vi "PDF Welding.vi"(0 "configuration file path":path caption="配置文件的路径", 1 "PDF Welding msic inf":T1) -> ()   [LabVIEW 2018]
uses:
  Ctl.xio/PDF Welding msic ctl.ctl
  SubVIS.xio/DataSocket/DataSocket_Tags.ctl
  Ctl.xio/part type.ctl
  SubVIS.xio/Creat Write List VI's/DefCtrl/Station.ctl
  SubVIS.xio/DataSocket/Write PLC Vars/Write Bool Var in.vi
  <vilib>/Utility/file.llb/Read From Spreadsheet File (string).vi
  SubVIS.xio/DataSocket/Write PLC Vars/Write String Var in.vi
  SubVIS.xio/DataSocket/Read PLC Vars/Read Bool Var.vi
  SubVIS.xio/DataSocket/Read PLC Vars/Read U32 Var.vi
  SubVIS.xio/DataSocket/Write PLC Vars/Write Dbl Var in.vi
  SubVIS.xio/Hopper car inf/Curing inf.vi
panel:
  in  "SQL information":string
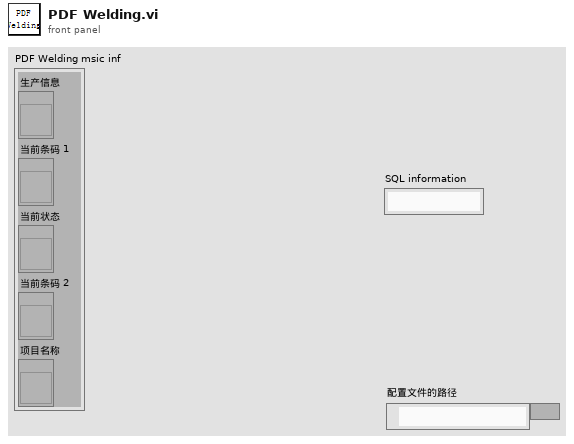
[diagram p1: front panel]
types:
  T1 = cluster{"生产信息":refnum<vi>, "当前条码 1":refnum<vi>, "当前状态":refnum<vi>, "当前条码 2":refnum<vi>, "项目名称":refnum<vi>}
  T2 = typedef "Station.ctl" = enum16{"粗切工位", "热处理工位", "精切工位", "PDF焊接工位", "打凹点预载力工位", "收卷工位", "EOL工位"}
  T3 = typedef "PDF Welding msic ctl.ctl" = cluster{"configuration file path":path, "DsOut":T4[], "Hopper car information":cluster{"Hopper car code":string, "Hopper car No":string, "plate No":string}, "pallet.produced number":i32, "SQL information":string, "Serial number":i32, "database path":path, "PDF Welding msic inf":cluster{"生产信息":refnum<vi>, "当前条码 1":refnum<vi>, "当前状态":refnum<vi>, "当前条码 2":refnum<vi>, "项目名称":refnum<vi>}, "Heating process parameters":cluster{"heating start":string, "heating finish":string, "Heating time use":u32}, "part type":T5, "Inlet temperature database":string[], "Outlet temperature database":string[], "Inlet temperature buffer":i32[], "Outlet temperature buffer":i32[], "PDF start time":string, "PDF finish time":string, "BarCode1":string, "BarCode2":string, "scanner resource name out":refnum<visa-resource-name>, "scanner coms or ip":string, "Outlet pressure buffer":i32[], "Outlet pressure database":string[], "scanner ip ID":refnum<k5>}
  T4 = typedef "DataSocket_Tags.ctl" = cluster{"Ds ID":refnum<k13>, "Tag":string}
  T5 = typedef "part type.ctl" = cluster{"Part type":string, "Material code":string, "Part number":string, "Supplier code":string, "Line code":string, "Customer code":string, "Color code":string, "Upper limit":i32, "Temperature":string, "Tot time":string, "EOL stations":string}
  T6 = cluster{"Hopper car code":string, "Hopper car No":string, "plate No":string}
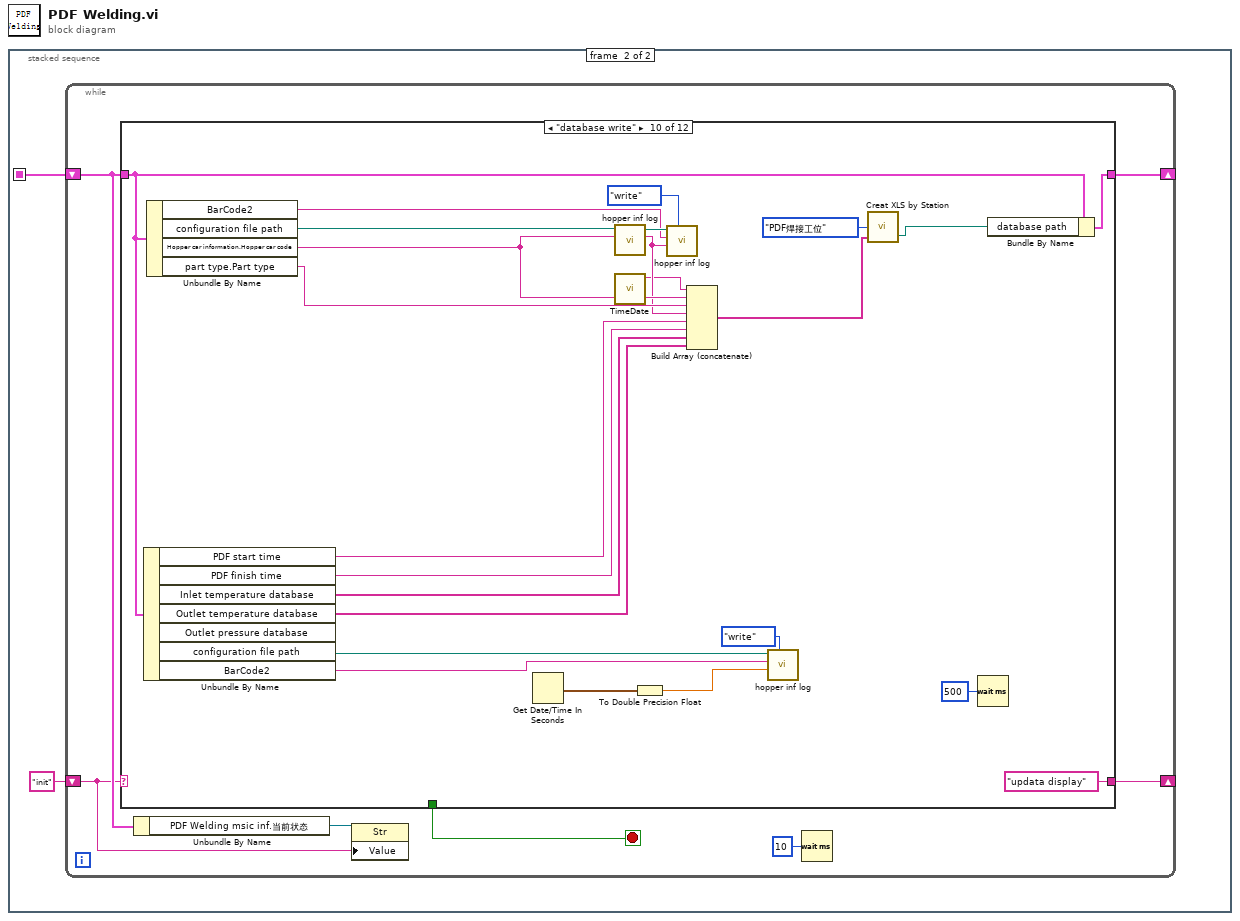
[diagram p0: block diagram]
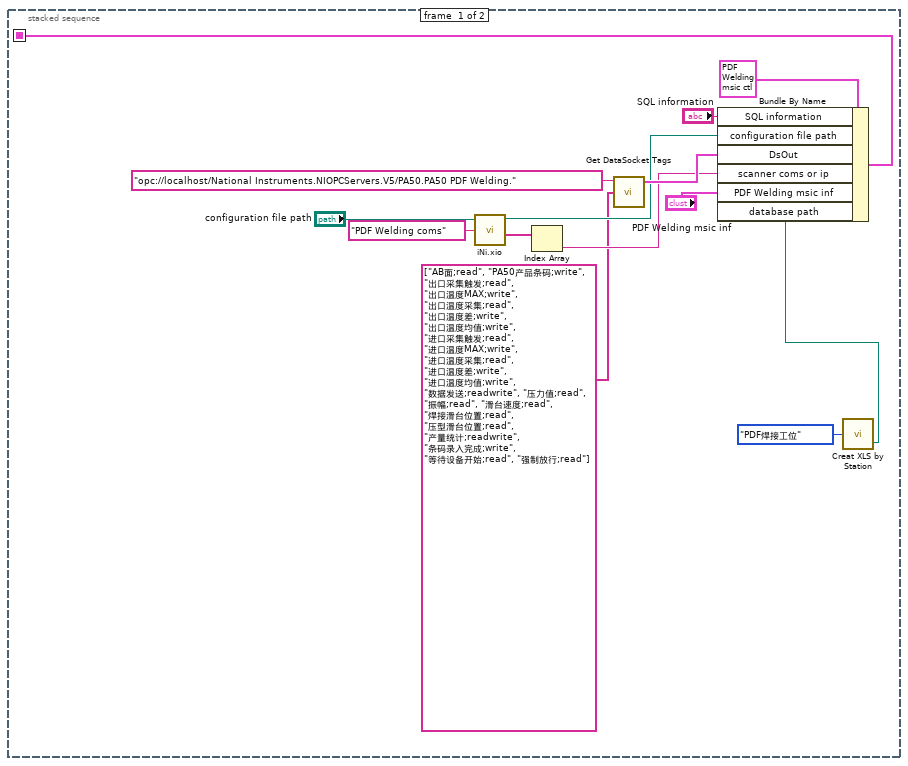
[diagram p2: hidden frame]
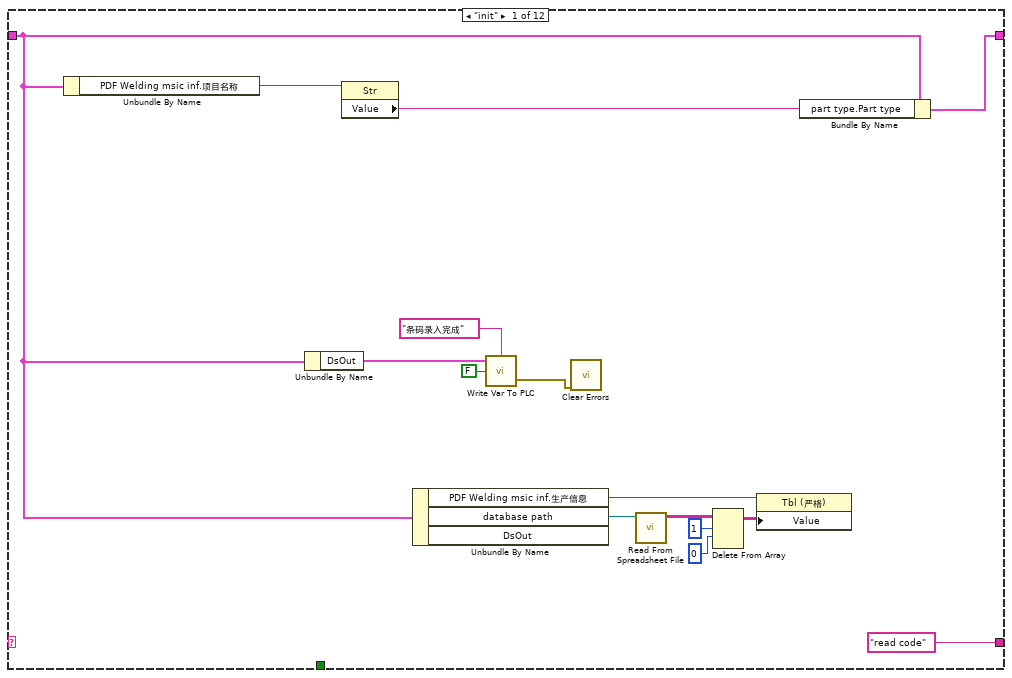
[diagram p3: hidden frame]
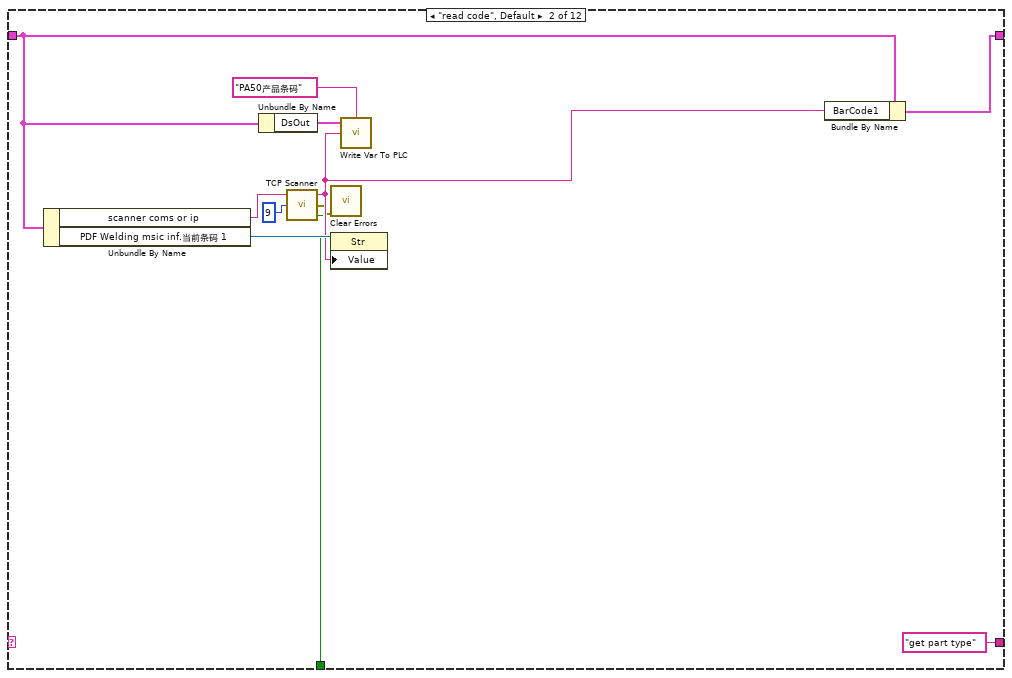
[diagram p4: hidden frame]
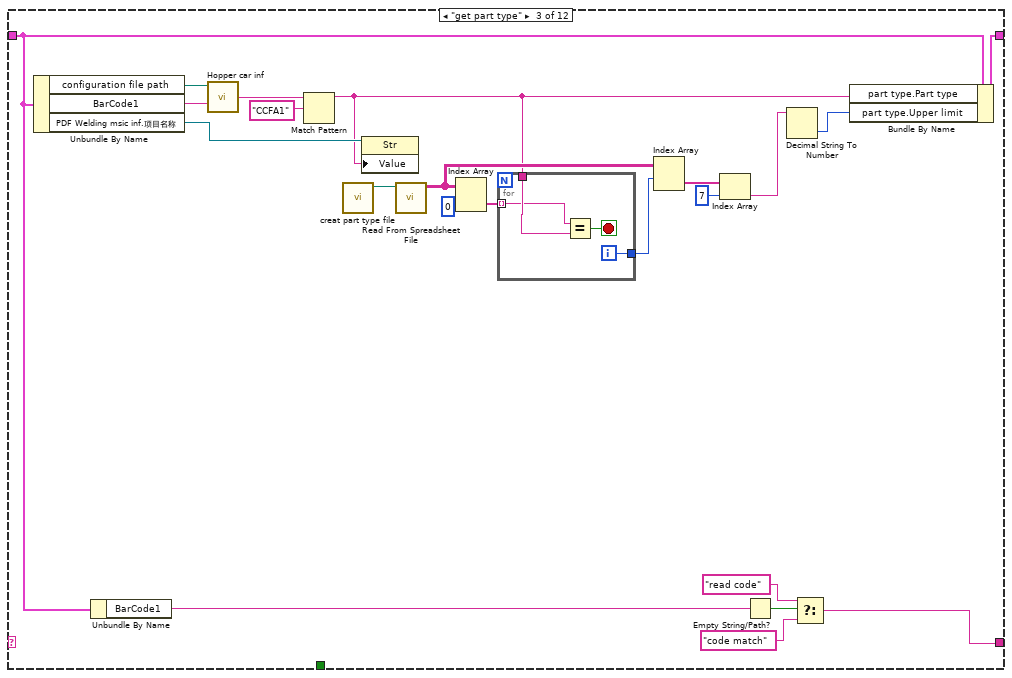
[diagram p5: hidden frame]
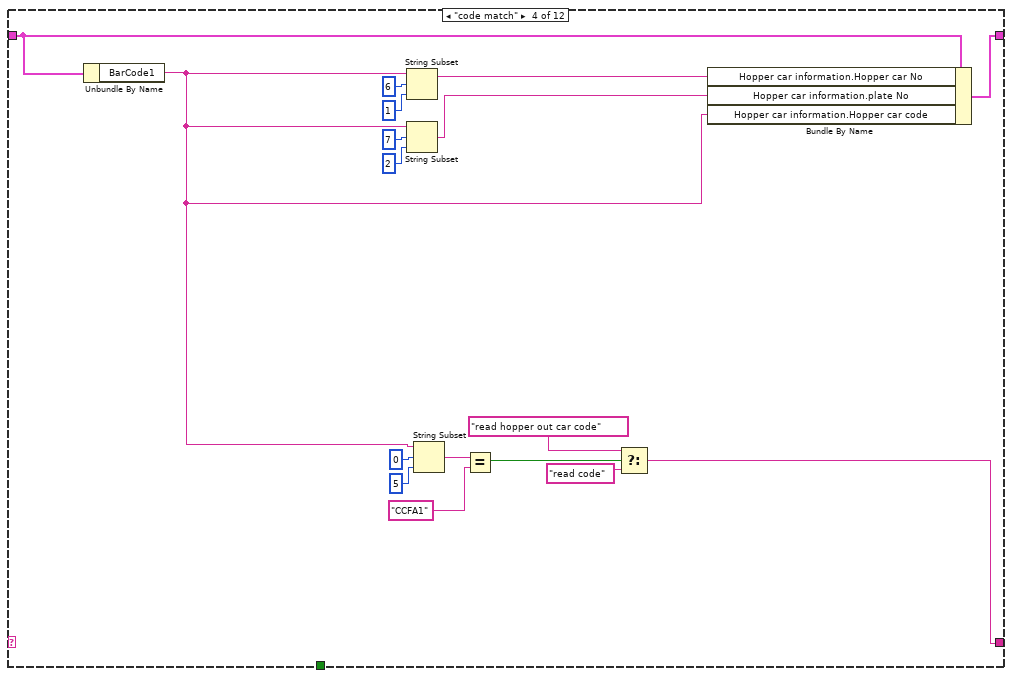
[diagram p6: hidden frame]
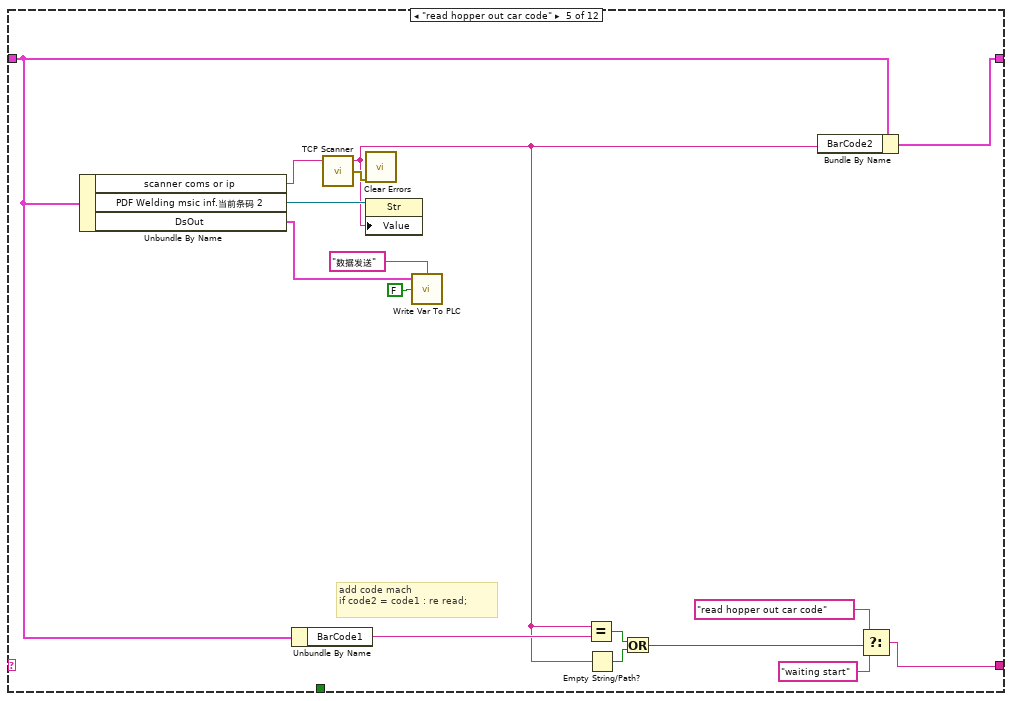
[diagram p7: hidden frame]
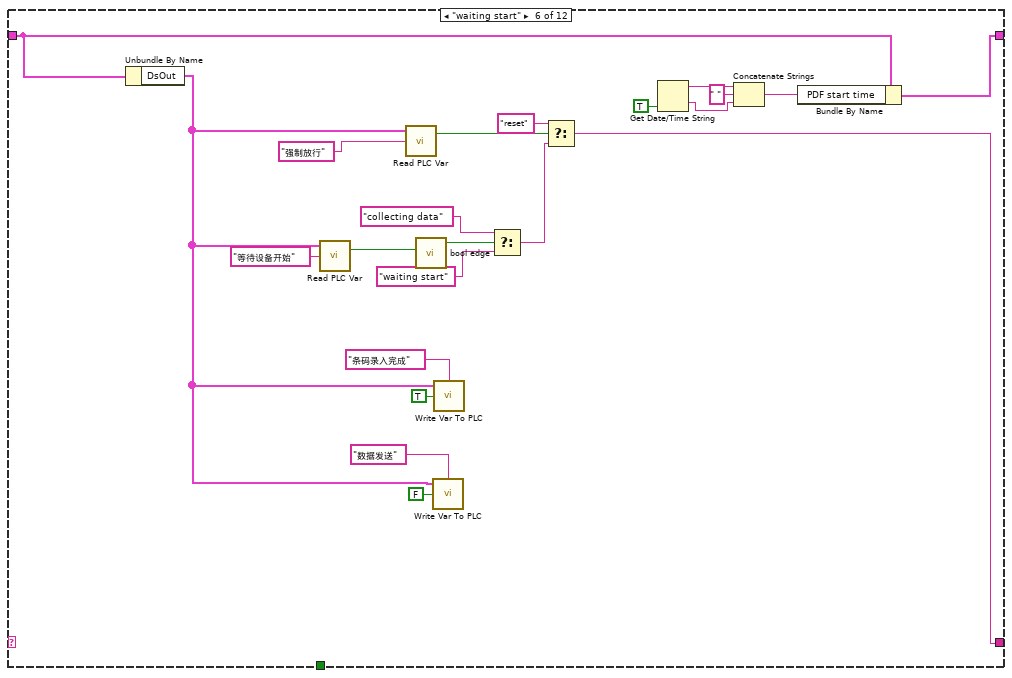
[diagram p8: hidden frame]
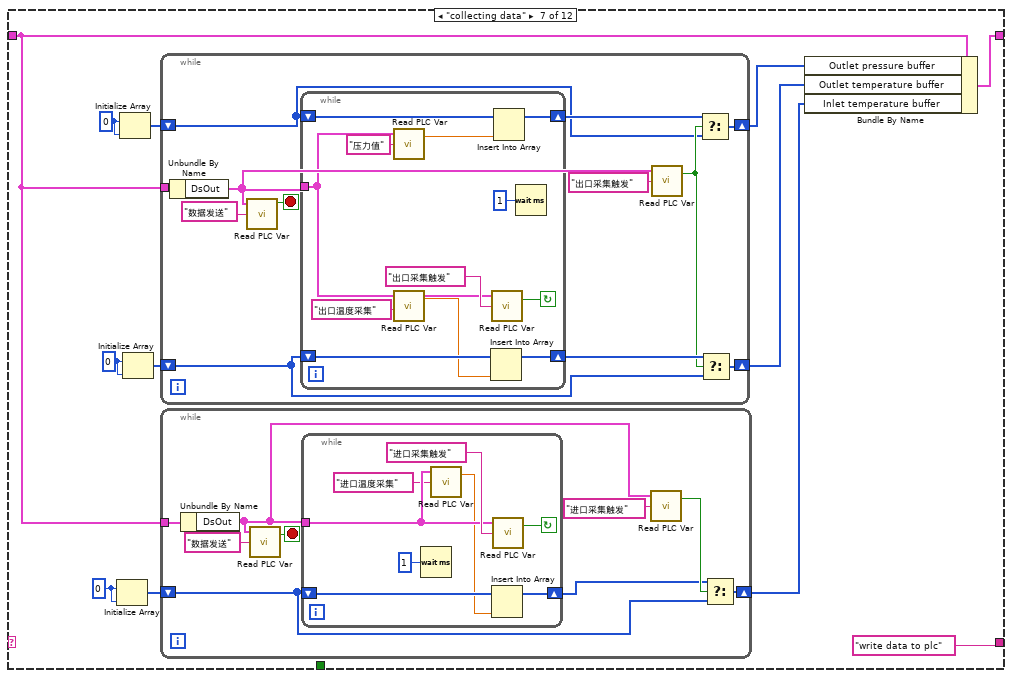
[diagram p9: hidden frame]
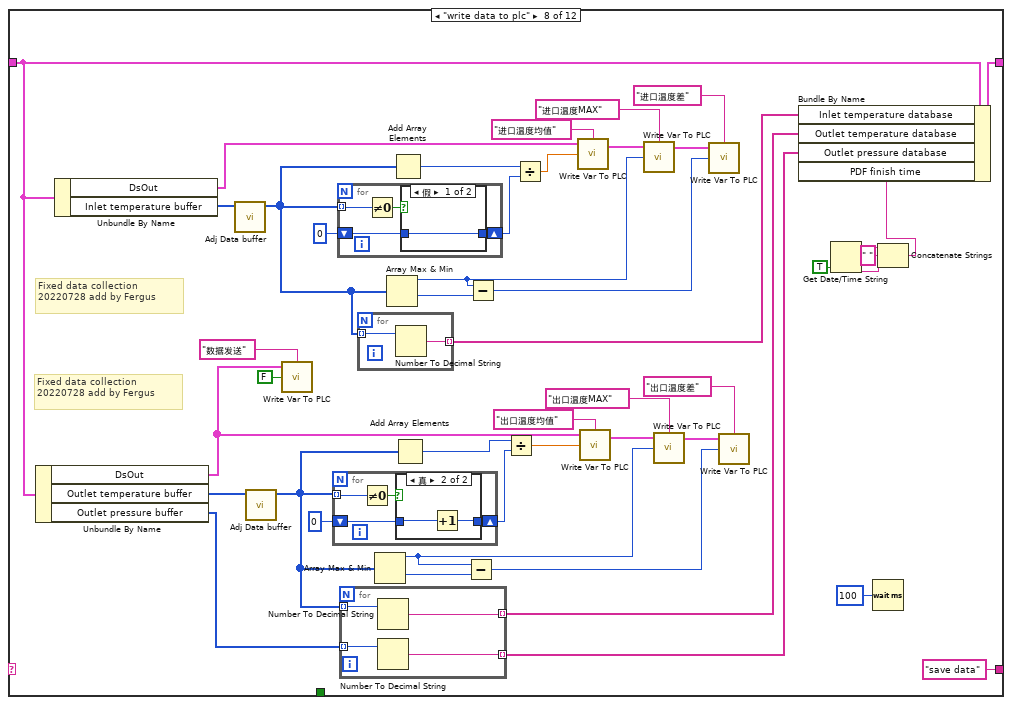
[diagram p10: hidden frame]
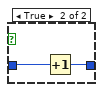
[diagram p12: hidden frame]
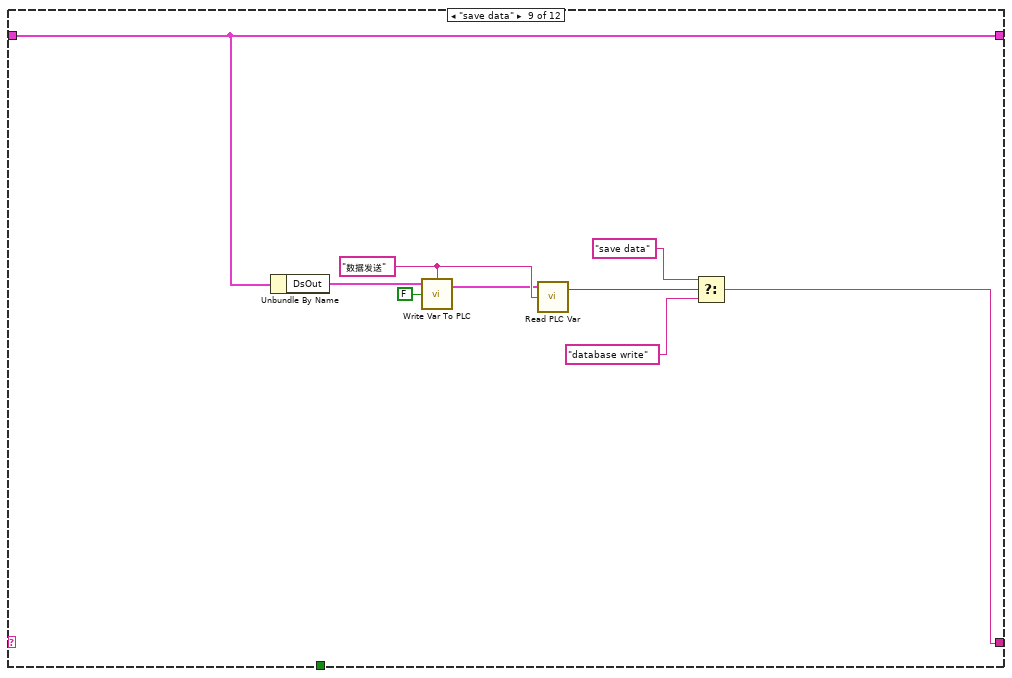
[diagram p13: hidden frame]
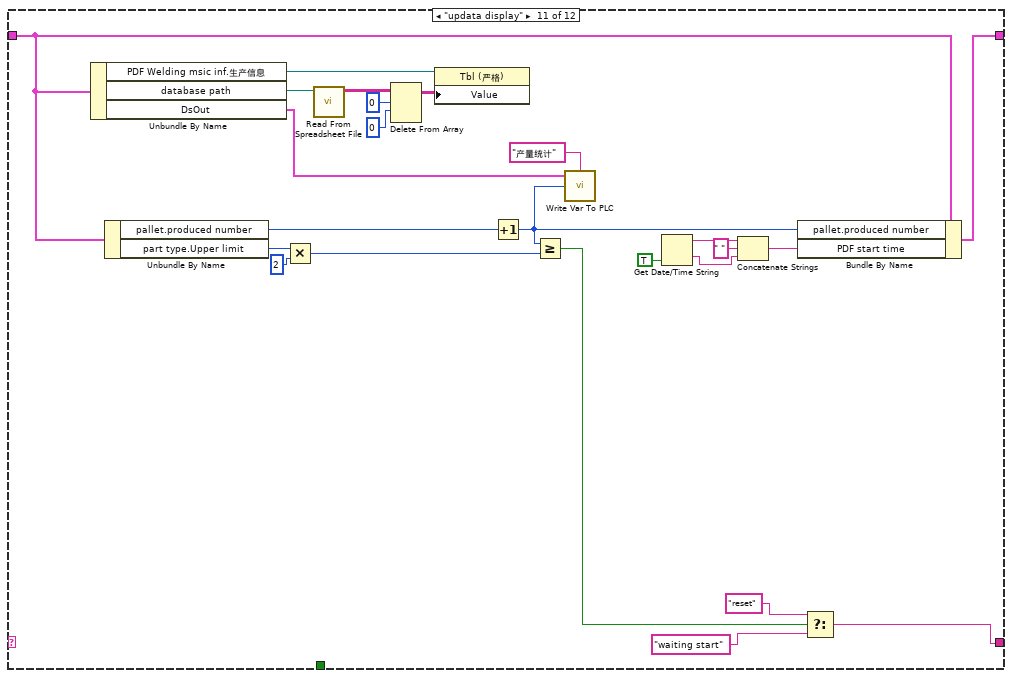
[diagram p14: hidden frame]
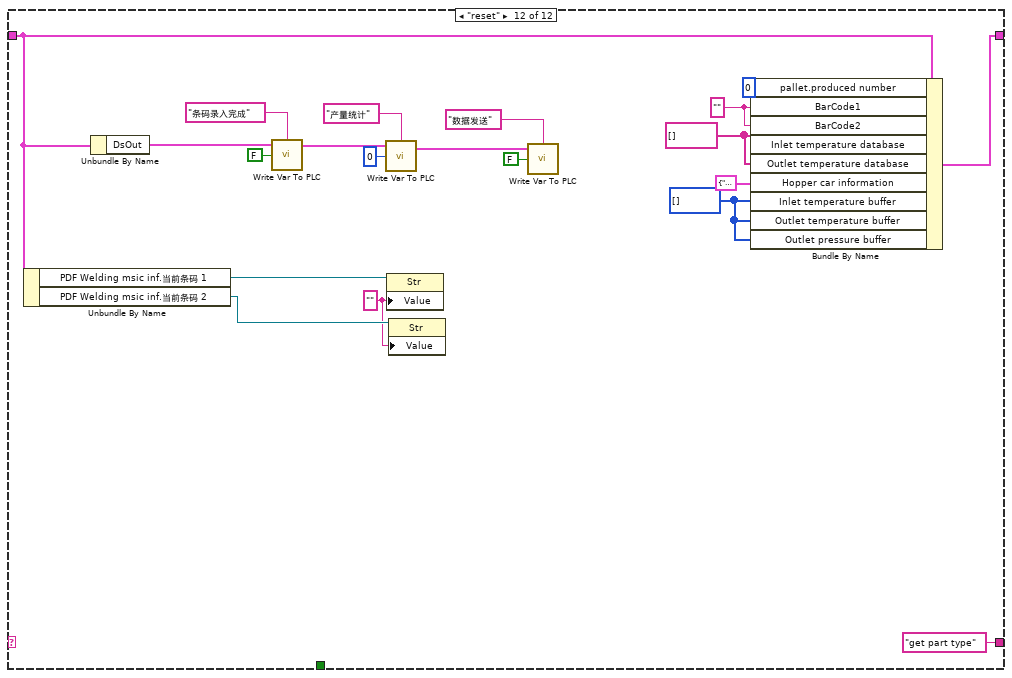
[diagram p15: hidden frame]
diagram:
  n1 = stacked-sequence {
    seq-local: [w3 _] -> [_ w15]
    frame #0 {
      n2 = call "iNi.xio.vi"("configuration file path"="configuration file path", "Sections"="PDF Welding coms") -> ("configuration file path"=w13:path, "Values"=w11:string[])  [unwired: 1 in, 3 out]
      n3 = Index Array(array=w11) -> (element=w10:string)  [unwired: 1 in]
      n4 = call "Get DataSocket Tags.vi"("All Tags"=string[] ["AB面;read", "PA50产品条码;write", "出口采集触发;read", "出口温度MAX;write", "出口温度采集;read", "出口温度差;write", "出口温度均值;write", "进口采集触发;read", "进口温度MAX;write", "进口温度采集;read", "进口温度差;write", "进口温度均值;write", "数据发送;readwrite", "压力值;read", "振幅;read", "滑台速度;read", "焊接滑台位置;read", "压型滑台位置;read", "产量统计;readwrite", "条码录入完成;write", "等待设备开始;read", "强制放行;read"], "URL"="opc://localhost/National Instruments.NIOPCServers.V5/PA50.PA50 PDF Welding.") -> ("DsOut"=w14:T4[])  [unwired: 3 in]
      n5 = call "Creat XLS by Station.vi"("staiton"=Station."PDF焊接工位") -> ("new file path (Not A Path if cancelled)"=w1:path)  [unwired: 5 in]
      n6 = Bundle By Name(cluster=T3 {"configuration file path"=path "", "DsOut"=[], "Hopper car information"={"Hopper car code"="", "Hopper car No"="", "plate No"=""}, "pallet.produced number"=0, "SQL information"="", "Serial number"=0, "database path"=path "", "PDF Welding msic inf"={"生产信息"=refnum, "当前条码 1"=refnum, "当前状态"=refnum, "当前条码 2"=refnum, "项目名称"=refnum}, "Heating process parameters"={"heating start"="", "heating finish"="", "Heating time use"=0}, "part type"={"Part type"="", "Material code"="", "Part number"="", "Supplier code"="", "Line code"="", "Customer code"="", "Color code"="", "Upper limit"=0, "Temperature"="", "Tot time"="", "EOL stations"=""}, "Inlet temperature database"=[], "Outlet temperature database"=[], "Inlet temperature buffer"=[], "Outlet temperature buffer"=[], "PDF start time"="", "PDF finish time"="", "BarCode1"="", "BarCode2"="", "scanner resource name out"="", "scanner coms or ip"="", "Outlet pressure buffer"=[], "Outlet pressure database"=[], "scanner ip ID"=refnum} ("PDF Welding msic ctl"), "SQL information"="SQL information", "configuration file path"=w13, "DsOut"=w14, "scanner coms or ip"=w10, "PDF Welding msic inf"="PDF Welding msic inf", "database path"=w1) -> (w3:T3)
    }
    frame #1 {
      n7 = while {
        shift-right: [w23] -> _
        shift-left: w15 -> [w19]
        shift-right: [w22] -> _
        shift-left: "init" ("event") -> [w18]
        stop <- w17 stop-if-true
        n8 = case shown="\"database write\"" w18 {
          tunnel: w19 -> [w25 w46 w54 w78 w98 w111 w131 w199 w256 w279 w296 w315]
          tunnel: [w38 w49 w71 w86 w107 w109 w142 w200 w256 w280 w295 w324] -> w23
          tunnel: ["read code" "get part type" ("f") w58 w85 w103 w122 "write data to plc" ("f") "save data" ("f") w249 "updata display" ("f") w291 "get part type" ("f")] -> w22
          tunnel: [_ w39 _ _ _ _ _ _ _ _ _ _] -> w17
          frame "init" {
            n9 = Unbundle By Name(w25) -> ("PDF Welding msic inf.项目名称"=w37:refnum<vi>)
            n10 = Unbundle By Name(w25) -> ("DsOut"=w34:T4[])
            n11 = property class="Str"(reference=w37) -> ("Value"=w36:string)  [unwired: 1 in, 2 out]
            n12 = Unbundle By Name(w25) -> ("PDF Welding msic inf.生产信息"=w31:refnum<vi>, "database path"=w30:path)  [unwired: 1 out]
            n13 = call-poly "Write Var To PLC.vi"("Tag IN"="条码录入完成", "Bool Var in"=FALSE, "Ds PLCTags IN"=w34) -> ("error out"=w24:errorcluster)  [unwired: 1 in, 1 out]
            n14 = call <vilib>:"Clear Errors.vi"("error in (no error)"=w24) -> ()  [unwired: 5 in, 2 out]
            n15 = call-poly <vilib>:"Read From Spreadsheet File.vi"("file path (dialog if empty)"=w30) -> ("all rows"=w29:string[][])  [unwired: 6 in, 4 out]
            n16 = Delete From Array(array=w29, length=1 ("长度"), index (row)=0 ("索引 (行)")) -> (array with subset deleted=w26:string[][])  [unwired: 1 in, 1 out]
            n17 = property class="Tbl (严格)"(reference=w31, "Value"=w26) -> ()  [unwired: 1 in, 2 out]
            n18 = Bundle By Name(cluster=w25, "part type.Part type"=w36) -> (w38:T3)
          }
          frame "read code", Default {
            n19 = Unbundle By Name(w46) -> ("scanner coms or ip"=w42:string, "PDF Welding msic inf.当前条码 1"=w48:refnum<vi>)
            n20 = Unbundle By Name(w46) -> ("DsOut"=w45:T4[])
            n21 = call "TCP Scanner.vi"("byte of read(9)"=9 ("读取的字节"), "ip"=w42) -> ("status"=w39:bool, "错误输出"=w40:errorcluster, "Barcode"=w44:string)  [unwired: 1 in]
            n22 = call <vilib>:"Clear Errors.vi"("error in (no error)"=w40) -> ()  [unwired: 5 in, 2 out]
            n23 = property class="Str"(reference=w48, "Value"=w44) -> ()  [unwired: 1 in, 2 out]
            n24 = call-poly "Write Var To PLC.vi"("Tag IN"="PA50产品条码", "String Var in"=w44, "Ds PLCTags IN"=w45) -> ()  [unwired: 1 in, 2 out]
            n25 = Bundle By Name(cluster=w46, "BarCode1"=w44) -> (w49:T3)
          }
          frame "get part type" {
            n26 = Unbundle By Name(w54) -> ("configuration file path"=w56:path, "BarCode1"=w55:string, "PDF Welding msic inf.项目名称"=w53:refnum<vi>)
            n27 = Unbundle By Name(w54) -> ("BarCode1"=w57:string)
            n28 = call "Hopper car inf.vi"("key"=w55, "path in"=w56) -> ("value out"=w52:string)  [unwired: 8 in, 1 out]
            n29 = Match Pattern(string=w52, regular expression="CCFA1" ("正则表达式")) -> (before substring=w50:string)  [unwired: 1 in, 3 out]
            n30 = call "creat part type file.vi"() -> ("new file path (Not A Path if cancelled)"=w62:path)  [unwired: 11 in]
            n31 = property class="Str"(reference=w53, "Value"=w50) -> ()  [unwired: 1 in, 2 out]
            n32 = call-poly <vilib>:"Read From Spreadsheet File.vi"("file path (dialog if empty)"=w62) -> ("all rows"=w67:string[][])  [unwired: 6 in, 4 out]
            n33 = Index Array(array=w67, index (col)=0 ("禁用的索引 (列)")) -> (element=w69:string[])  [unwired: 1 in]
            n34 = for {
              tunnel: w69 -> [w72] mode=indexing
              tunnel: [w74] -> w66
              tunnel: w50 -> [w73]
              i -> [w74]
              stop <- w75 stop-if-true
              n35 = Equal?(x=w72, y=w73) -> (x = y?=w75:bool)
            }
            n36 = Index Array(array=w67, index (row)=w66) -> (element=w65:string[])  [unwired: 1 in]
            n37 = Index Array(array=w65, index=7 ("索引")) -> (element=w64:string)
            n38 = Empty String/Path?(string/path=w57) -> (empty?=w61:bool)
            n39 = Decimal String To Number(string=w64) -> (number=w63:i32)  [unwired: 2 in, 1 out]
            n40 = Select(t="read code", s=w61, f="code match") -> (s? t:f=w58:string)
            n41 = Bundle By Name(cluster=w54, "part type.Part type"=w50, "part type.Upper limit"=w63) -> (w71:T3)
          }
          frame "code match" {
            n42 = Unbundle By Name(w78) -> ("BarCode1"=w77:string)
            n43 = String Subset(string=w77, offset (0)=6 ("偏移量(0)"), length (rest)=1 ("长度（剩余）")) -> (substring=w80:string)
            n44 = String Subset(string=w77, offset (0)=7 ("偏移量(0)"), length (rest)=2 ("长度（剩余）")) -> (substring=w81:string)
            n45 = String Subset(string=w77, offset (0)=0 ("偏移量(0)"), length (rest)=5 ("长度（剩余）")) -> (substring=w82:string)
            n46 = Equal?(x=w82, y="CCFA1") -> (x = y?=w76:bool)
            n47 = Select(t="read hopper out car code" ("event"), s=w76, f="read code" ("event")) -> (s? t:f=w85:string)
            n48 = Bundle By Name(cluster=w78, "Hopper car information.Hopper car No"=w80, "Hopper car information.plate No"=w81, "Hopper car information.Hopper car code"=w77) -> (w86:T3)
          }
          frame "read hopper out car code" {
            # "add code mach\nif code2 = code1 : re read;"
            n49 = Unbundle By Name(w98) -> ("scanner coms or ip"=w108:string, "PDF Welding msic inf.当前条码 2"=w106:refnum<vi>, "DsOut"=w99:T4[])
            n50 = Unbundle By Name(w98) -> ("BarCode1"=w97:string)
            n51 = call "TCP Scanner.vi"("ip"=w108) -> ("错误输出"=w102:errorcluster, "Barcode"=w96:string)  [unwired: 2 in, 1 out]
            n52 = call <vilib>:"Clear Errors.vi"("error in (no error)"=w102) -> ()  [unwired: 5 in, 2 out]
            n53 = property class="Str"(reference=w106, "Value"=w96) -> ()  [unwired: 1 in, 2 out]
            n54 = call-poly "Write Var To PLC.vi"("Tag IN"="数据发送", "Bool Var in"=FALSE, "Ds PLCTags IN"=w99) -> ()  [unwired: 1 in, 2 out]
            n55 = Equal?(x=w96, y=w97) -> (x = y?=w95:bool)
            n56 = Empty String/Path?(string/path=w96) -> (empty?=w94:bool)
            n57 = Or(x=w95, y=w94) -> (x .or. y?=w93:bool)
            n58 = Bundle By Name(cluster=w98, "BarCode2"=w96) -> (w107:T3)
            n59 = Select(t="read hopper out car code" ("f"), s=w93, f="waiting start") -> (s? t:f=w103:string)
          }
          frame "waiting start" {
            n60 = Unbundle By Name(w111) -> ("DsOut"=w116:T4[])
            n61 = call-poly "Read PLC Var.vi"("Tag IN"="等待设备开始", "Ds PLCTags IN"=w116) -> ("Bool Var out"=w129:bool)  [unwired: 1 in, 1 out]
            n62 = call-poly "Read PLC Var.vi"("Tag IN"="强制放行", "Ds PLCTags IN"=w116) -> ("Bool Var out"=w124:bool)  [unwired: 1 in, 1 out]
            n63 = call "bool edge.vi"("bool in"=w129) -> ("false-true"=w128:bool)  [unwired: 6 in, 1 out]
            n64 = call-poly "Write Var To PLC.vi"("Tag IN"="数据发送", "Bool Var in"=FALSE, "Ds PLCTags IN"=w116) -> ()  [unwired: 1 in, 2 out]
            n65 = call-poly "Write Var To PLC.vi"("Tag IN"="条码录入完成", "Bool Var in"=TRUE, "Ds PLCTags IN"=w116) -> ()  [unwired: 1 in, 2 out]
            n66 = Select(t="collecting data" ("f"), s=w128, f="waiting start") -> (s? t:f=w123:string)
            n67 = Select(t="reset" ("f"), s=w124, f=w123) -> (s? t:f=w122:string)
            n68 = Get Date/Time String(want seconds? (F)=TRUE ("需要秒？(F)")) -> (date string=w115:string, time string=w113:string)  [unwired: 2 in]
            n69 = Concatenate Strings(w115, " " ("字符串"), w113) -> (w110:string)
            n70 = Bundle By Name(cluster=w111, "PDF start time"=w110) -> (w109:T3)
          }
          frame "collecting data" {
            w134 = 0 ("维数大小")
            w136 = 0 ("维数大小")
            w139 = 0 ("维数大小")
            n71 = Initialize Array(w136, w136) -> (w135:i32[])
            n72 = Initialize Array(w134, w134) -> (w133:i32[])
            n73 = Initialize Array(w139, w139) -> (w138:i32[])
            n74 = while {
              tunnel: w131 -> [w171]
              shift-right: [w164] -> w137
              shift-left: w138 -> [w165]
              shift-right: [w163] -> w132
              shift-left: w133 -> [w160]
              stop <- w169 stop-if-true
              n75 = Unbundle By Name(w171) -> ("DsOut"=w168:T4[])
              n76 = call-poly "Read PLC Var.vi"("Tag IN"="数据发送", "Ds PLCTags IN"=w168) -> ("Bool Var out"=w169:bool)  [unwired: 1 in, 1 out]
              n77 = while {
                tunnel: w168 -> [w176]
                shift-right: [w178] -> w166
                shift-left: w165 -> [w180]
                shift-right: [w172] -> w161
                shift-left: w160 -> [w173]
                stop <- w183 continue-if-true
                n78 = call-poly "Read PLC Var.vi"("Tag IN"="压力值", "Ds PLCTags IN"=w176) -> ("U32 Var out"=w174:dbl)  [unwired: 1 in, 1 out]
                n79 = call-poly "Read PLC Var.vi"("Tag IN"="出口温度采集", "Ds PLCTags IN"=w176) -> ("U32 Var out"=w179:dbl)  [unwired: 1 in, 1 out]
                n80 = Insert Into Array(array=w180, new element=w179) -> (w178:i32[])  [unwired: 1 in]
                n81 = call-poly "Read PLC Var.vi"("Tag IN"="出口采集触发", "Ds PLCTags IN"=w176) -> ("Bool Var out"=w183:bool)  [unwired: 1 in, 1 out]
                n82 = Insert Into Array(array=w173, new element=w174) -> (w172:i32[])  [unwired: 1 in]
                n83 = Wait (ms)(milliseconds to wait=u32 1 ("等待时间（毫秒）")) -> ()  [unwired: 1 out]
              }
              n84 = call-poly "Read PLC Var.vi"("Tag IN"="出口采集触发", "Ds PLCTags IN"=w168) -> ("Bool Var out"=w162:bool)  [unwired: 1 in, 1 out]
              n85 = Select(t=w161, s=w162, f=w160) -> (s? t:f=w163:i32[])
              n86 = Select(t=w166, s=w162, f=w165) -> (s? t:f=w164:i32[])
            }
            n87 = while {
              tunnel: w131 -> [w151]
              shift-right: [w146] -> w141
              shift-left: w135 -> [w143]
              stop <- w149 stop-if-true
              n88 = Unbundle By Name(w151) -> ("DsOut"=w148:T4[])
              n89 = call-poly "Read PLC Var.vi"("Tag IN"="数据发送", "Ds PLCTags IN"=w148) -> ("Bool Var out"=w149:bool)  [unwired: 1 in, 1 out]
              n90 = while {
                tunnel: w148 -> [w157]
                shift-right: [w153] -> w144
                shift-left: w143 -> [w155]
                stop <- w159 continue-if-true
                n91 = Wait (ms)(milliseconds to wait=u32 1 ("等待时间（毫秒）")) -> ()  [unwired: 1 out]
                n92 = call-poly "Read PLC Var.vi"("Tag IN"="进口温度采集", "Ds PLCTags IN"=w157) -> ("U32 Var out"=w154:dbl)  [unwired: 1 in, 1 out]
                n93 = Insert Into Array(array=w155, new element=w154) -> (w153:i32[])  [unwired: 1 in]
                n94 = call-poly "Read PLC Var.vi"("Tag IN"="进口采集触发", "Ds PLCTags IN"=w157) -> ("Bool Var out"=w159:bool)  [unwired: 1 in, 1 out]
              }
              n95 = call-poly "Read PLC Var.vi"("Tag IN"="进口采集触发", "Ds PLCTags IN"=w148) -> ("Bool Var out"=w145:bool)  [unwired: 1 in, 1 out]
              n96 = Select(t=w144, s=w145, f=w143) -> (s? t:f=w146:i32[])
            }
            n97 = Bundle By Name(cluster=w131, "Outlet pressure buffer"=w132, "Outlet temperature buffer"=w137, "Inlet temperature buffer"=w141) -> (w142:T3)
          }
          frame "write data to plc" {
            # "Fixed data collection\n20220728 add by Fergus"
            # "Fixed data collection\n20220728 add by Fergus"
            n98 = Unbundle By Name(w199) -> ("DsOut"=w196:T4[], "Outlet temperature buffer"=w185:i32[], "Outlet pressure buffer"=w190:i32[])
            n99 = Unbundle By Name(w199) -> ("DsOut"=w224:T4[], "Inlet temperature buffer"=w187:i32[])
            n100 = call "Adj Data buffer.vi"("data buffer"=w187) -> ("data buffer out"=w186:i32[])  [unwired: 10 in]
            n101 = call "Adj Data buffer.vi"("data buffer"=w185) -> ("data buffer out"=w184:i32[])  [unwired: 10 in]
            n102 = call-poly "Write Var To PLC.vi"("Tag IN"="数据发送", "Bool Var in"=FALSE, "Ds PLCTags IN"=w196) -> ()  [unwired: 1 in, 2 out]
            n103 = for {
              tunnel: w184 -> [w238] mode=indexing
              shift-right: [w235] -> w219
              shift-left: 0 -> [w236]
              n104 = Not Equal To 0?(x=w238) -> (x != 0?=w237:bool)
              n105 = case shown="真" w237 {
                tunnel: w236 -> [w239 w240]
                tunnel: [w239 w241] -> w235
                frame False {
                }
                frame True {
                  n106 = Increment(x=w240) -> (x+1=w241:i32)
                }
              }
            }
            n107 = for {
              tunnel: w186 -> [w245] mode=indexing
              shift-right: [w242] -> w226
              shift-left: 0 -> [w243]
              n108 = Not Equal To 0?(x=w245) -> (x != 0?=w244:bool)
              n109 = case shown="假" w244 {
                tunnel: w243 -> [w246 w247]
                tunnel: [w246 w248] -> w242
                frame False {
                }
                frame True {
                  n110 = Increment(x=w247) -> (x+1=w248:i32)
                }
              }
            }
            n111 = for {
              tunnel: w184 -> [w232] mode=indexing
              tunnel: [w230] -> w202 mode=indexing
              tunnel: w190 -> [w231] mode=indexing
              tunnel: [w229] -> w188 mode=indexing
              n112 = Number To Decimal String(number=w232) -> (decimal integer string=w230:string)  [unwired: 1 in]
              n113 = Number To Decimal String(number=w231) -> (decimal integer string=w229:string)  [unwired: 1 in]
            }
            n114 = for {
              tunnel: w186 -> [w234] mode=indexing
              tunnel: [w233] -> w203 mode=indexing
              n115 = Number To Decimal String(number=w234) -> (decimal integer string=w233:string)  [unwired: 1 in]
            }
            n116 = Array Max & Min(array=w184) -> (max value=w206:i32, min value=w205:i32)  [unwired: 2 out]
            n117 = Array Max & Min(array=w186) -> (max value=w214:i32, min value=w217:i32)  [unwired: 2 out]
            n118 = Add Array Elements(numeric array=w186) -> (sum=w225:i32)
            n119 = Add Array Elements(numeric array=w184) -> (sum=w220:i32)
            n120 = Subtract(x=w206, y=w205) -> (x-y=w204:i32)
            n121 = Subtract(x=w214, y=w217) -> (x-y=w211:i32)
            n122 = Divide(x=w220, y=w219) -> (x/y=w218:dbl)
            n123 = Divide(x=w225, y=w226) -> (x/y=w222:dbl)
            n124 = call-poly "Write Var To PLC.vi"("Tag IN"="进口温度均值", "Dbl Var in"=w222, "Ds PLCTags IN"=w224) -> ("Ds PLCTags OUT"=w216:T4[])  [unwired: 1 in, 1 out]
            n125 = call-poly "Write Var To PLC.vi"("Tag IN"="出口温度均值", "Dbl Var in"=w218, "Ds PLCTags IN"=w196) -> ("Ds PLCTags OUT"=w207:T4[])  [unwired: 1 in, 1 out]
            n126 = call-poly "Write Var To PLC.vi"("Tag IN"="进口温度MAX", "Dbl Var in"=w214, "Ds PLCTags IN"=w216) -> ("Ds PLCTags OUT"=w213:T4[])  [unwired: 1 in, 1 out]
            n127 = call-poly "Write Var To PLC.vi"("Tag IN"="出口温度MAX", "Dbl Var in"=w206, "Ds PLCTags IN"=w207) -> ("Ds PLCTags OUT"=w209:T4[])  [unwired: 1 in, 1 out]
            n128 = call-poly "Write Var To PLC.vi"("Tag IN"="进口温度差", "Dbl Var in"=w211, "Ds PLCTags IN"=w213) -> ()  [unwired: 1 in, 2 out]
            n129 = call-poly "Write Var To PLC.vi"("Tag IN"="出口温度差", "Dbl Var in"=w204, "Ds PLCTags IN"=w209) -> ()  [unwired: 1 in, 2 out]
            n130 = Get Date/Time String(want seconds? (F)=TRUE ("需要秒？(F)")) -> (date string=w195:string, time string=w193:string)  [unwired: 2 in]
            n131 = Wait (ms)(milliseconds to wait=u32 100 ("等待时间（毫秒）")) -> ()  [unwired: 1 out]
            n132 = Concatenate Strings(w195, " " ("字符串"), w193) -> (w191:string)
            n133 = Bundle By Name(cluster=w199, "Inlet temperature database"=w203, "Outlet temperature database"=w202, "Outlet pressure database"=w188, "PDF finish time"=w191) -> (w200:T3)
          }
          frame "save data" {
            w254 = "数据发送" ("Tag IN")
            n134 = Unbundle By Name(w256) -> ("DsOut"=w255:T4[])
            n135 = call-poly "Write Var To PLC.vi"("Tag IN"=w254, "Bool Var in"=FALSE, "Ds PLCTags IN"=w255) -> ("Ds PLCTags OUT"=w253:T4[])  [unwired: 1 in, 1 out]
            n136 = call-poly "Read PLC Var.vi"("Tag IN"=w254, "Ds PLCTags IN"=w253) -> ("Bool Var out"=w252:bool)  [unwired: 1 in, 1 out]
            n137 = Select(t="save data" ("f"), s=w252, f="database write") -> (s? t:f=w249:string)
          }
          frame "database write" {
            n138 = Unbundle By Name(w279) -> ("PDF start time"=w275:string, "PDF finish time"=w274:string, "Inlet temperature database"=w273:string[], "Outlet temperature database"=w272:string[], "configuration file path"=w267:path, "BarCode2"=w264:string)  [unwired: 1 out]
            n139 = Unbundle By Name(w279) -> ("BarCode2"=w269:string, "configuration file path"=w278:path, "Hopper car information.Hopper car code"=w277:string, "part type.Part type"=w276:string)
            n140 = Get Date/Time In Seconds() -> (seconds since 1Jan1904=w266:timestamp)
            n141 = call-poly "hopper inf log.vi"("key"=w277, "path in"=w278) -> ("value out"=w268:string, "path out"=w271:path)  [unwired: 8 in]
            n142 = call "TimeDate.vi"() -> ("time_YMD"=w258:string)  [unwired: 10 in, 1 out]
            n143 = To Double Precision Float(number=w266) -> (double precision float=w265:dbl)
            n144 = call-poly "hopper inf log.vi"("write\\read（read)"=enum16{"read", "write"}."write" ("write\\read（read)"), "value"=w268, "key"=w269, "path in"=w271) -> ()  [unwired: 6 in, 2 out]
            n145 = Build Array (concatenate)(w258, w277, w276, w268, w275, w274, w273, w272) -> (w259:string[])
            n146 = call-poly "hopper inf log.vi"("write\\read（read)"=enum16{"read", "write"}."write" ("write\\read（read)"), "value in"=w265, "key"=w264, "path in"=w267) -> ()  [unwired: 6 in, 2 out]
            n147 = call "Creat XLS by Station.vi"("staiton"=Station."PDF焊接工位", "data in"=w259) -> ("new file path (Not A Path if cancelled)"=w260:path)  [unwired: 4 in]
            n148 = Wait (ms)(milliseconds to wait=u32 500 ("等待时间（毫秒）")) -> ()  [unwired: 1 out]
            n149 = Bundle By Name(cluster=w279, "database path"=w260) -> (w280:T3)
          }
          frame "updata display" {
            n150 = Unbundle By Name(w296) -> ("PDF Welding msic inf.生产信息"=w305:refnum<vi>, "database path"=w304:path, "DsOut"=w289:T4[])
            n151 = Unbundle By Name(w296) -> ("pallet.produced number"=w290:i32, "part type.Upper limit"=w299:i32)
            n152 = Multiply(x=w299, y=2) -> (x*y=w297:i32)
            n153 = call-poly <vilib>:"Read From Spreadsheet File.vi"("file path (dialog if empty)"=w304) -> ("all rows"=w303:string[][])  [unwired: 6 in, 4 out]
            n154 = Delete From Array(array=w303, length=0 ("长度"), index (row)=0 ("索引 (行)")) -> (array with subset deleted=w300:string[][])  [unwired: 1 in, 1 out]
            n155 = property class="Tbl (严格)"(reference=w305, "Value"=w300) -> ()  [unwired: 1 in, 2 out]
            n156 = Increment(x=w290) -> (x+1=w287:i32)
            n157 = Greater Or Equal?(x=w287, y=w297) -> (x >= y?=w294:bool)
            n158 = call-poly "Write Var To PLC.vi"("Tag IN"="产量统计", "Dbl Var in"=w287, "Ds PLCTags IN"=w289) -> ()  [unwired: 1 in, 2 out]
            n159 = Get Date/Time String(want seconds? (F)=TRUE ("需要秒？(F)")) -> (date string=w286:string, time string=w284:string)  [unwired: 2 in]
            n160 = Concatenate Strings(w286, " " ("字符串"), w284) -> (w282:string)
            n161 = Bundle By Name(cluster=w296, "pallet.produced number"=w287, "PDF start time"=w282) -> (w295:T3)
            n162 = Select(t="reset" ("f"), s=w294, f="waiting start") -> (s? t:f=w291:string)
          }
          frame "reset" {
            w312 = "" ("值")
            w319 = i32[] [] ("Inlet temperature buffer")
            w321 = string[] [] ("Database")
            w320 = "" ("BarCode")
            n163 = Unbundle By Name(w315) -> ("PDF Welding msic inf.当前条码 1"=w314:refnum<vi>, "PDF Welding msic inf.当前条码 2"=w313:refnum<vi>)
            n164 = Unbundle By Name(w315) -> ("DsOut"=w318:T4[])
            n165 = call-poly "Write Var To PLC.vi"("Tag IN"="条码录入完成", "Bool Var in"=FALSE, "Ds PLCTags IN"=w318) -> ("Ds PLCTags OUT"=w311:T4[])  [unwired: 1 in, 1 out]
            n166 = call-poly "Write Var To PLC.vi"("Tag IN"="产量统计", "Dbl Var in"=0, "Ds PLCTags IN"=w311) -> ("Ds PLCTags OUT"=w306:T4[])  [unwired: 1 in, 1 out]
            n167 = property class="Str"(reference=w314, "Value"=w312) -> ()  [unwired: 1 in, 2 out]
            n168 = property class="Str"(reference=w313, "Value"=w312) -> ()  [unwired: 1 in, 2 out]
            n169 = call-poly "Write Var To PLC.vi"("Tag IN"="数据发送", "Bool Var in"=FALSE, "Ds PLCTags IN"=w306) -> ()  [unwired: 1 in, 2 out]
            n170 = Bundle By Name(cluster=w315, "pallet.produced number"=0, "BarCode1"=w320, "BarCode2"=w320, "Inlet temperature database"=w321, "Outlet temperature database"=w321, "Hopper car information"=T6 {"Hopper car code"="", "Hopper car No"="", "plate No"=""}, "Inlet temperature buffer"=w319, "Outlet temperature buffer"=w319, "Outlet pressure buffer"=w319) -> (w324:T3)
          }
        }
        n171 = Unbundle By Name(w19) -> ("PDF Welding msic inf.当前状态"=w20:refnum<vi>)
        n172 = property class="Str"(reference=w20, "Value"=w18) -> ()  [unwired: 1 in, 2 out]
        n173 = Wait (ms)(milliseconds to wait=u32 10 ("等待时间（毫秒）")) -> ()  [unwired: 1 out]
      }
    }
  }
